vi "Save Data Single Station.vi"(5 "index":i32, 7 "Appliance Details":T1[](array[typedef]) {"Dryer"."Dryer Initial IMC Data"."Maximum Weight (lbf)" format="%03_6g"; "Dryer"."Dryer Initial IMC Data"."Average Weight (lbf)" format="%03_6g"; "Dryer"."Dryer Initial IMC Data"."Minimum Weight (lbf)" format="%03_6g"; "Dryer"."Dryer Initial IMC Data"."CEF (lbf/kWh)" format="%03_6g"; "Dryer"."Dryer Initial IMC Data"."Actual Final RMC (%)" format="%03_6g"; "Dryer"."Dryer Initial IMC Data"."Tolerance(%)" format="%0#_6g"; "Dryer"."Dryer Initial IMC Data"."Bone Dry Wt(lbs)" format="%03_6g"; "Dryer"."Dryer Initial IMC Data"."RMC (Desired %)" format="%0#_6g"; "Dryer"."Dryer Initial IMC Data"."Actual Initial RMC (%)" format="%03_6g"; "Dryer"."Dryer Initial IMC Data"."Measured IMC (lbs)" format="%0#_6g"}, 8 "Error In":errorcluster, 9 "File Locations in":T7, 10 "Data Array":string[][](array[string]), 11 "Log Data?":bool) -> (0 "Error Out":errorcluster, 2 "Saving":bool, 3 "File Locations out":T7)   [LabVIEW 2016]
uses:
  File Setup (Public)/Type Definition/Save File DOE File Path Control.ctl
  File Setup (Public)/Type Definition/Save File DOE Data Save Filepaths.ctl
  File Setup (Public)/Type Definition/Save File DISH Dishwasher Details.ctl
  <vilib>/Platform/fileVersionInfo.llb/FileVersionInformation.ctl
  Washer DOE/Type Definitions/DOE Appliance Common.ctl
  Custom Pallet Controls/Custom Pallet String.ctl
  File Setup (Public)/Type Definition/DPT IMC Data.ctl
  Washer DOE/Type Definitions/DOE Dryer Standard.ctl
  File Setup.lvlib
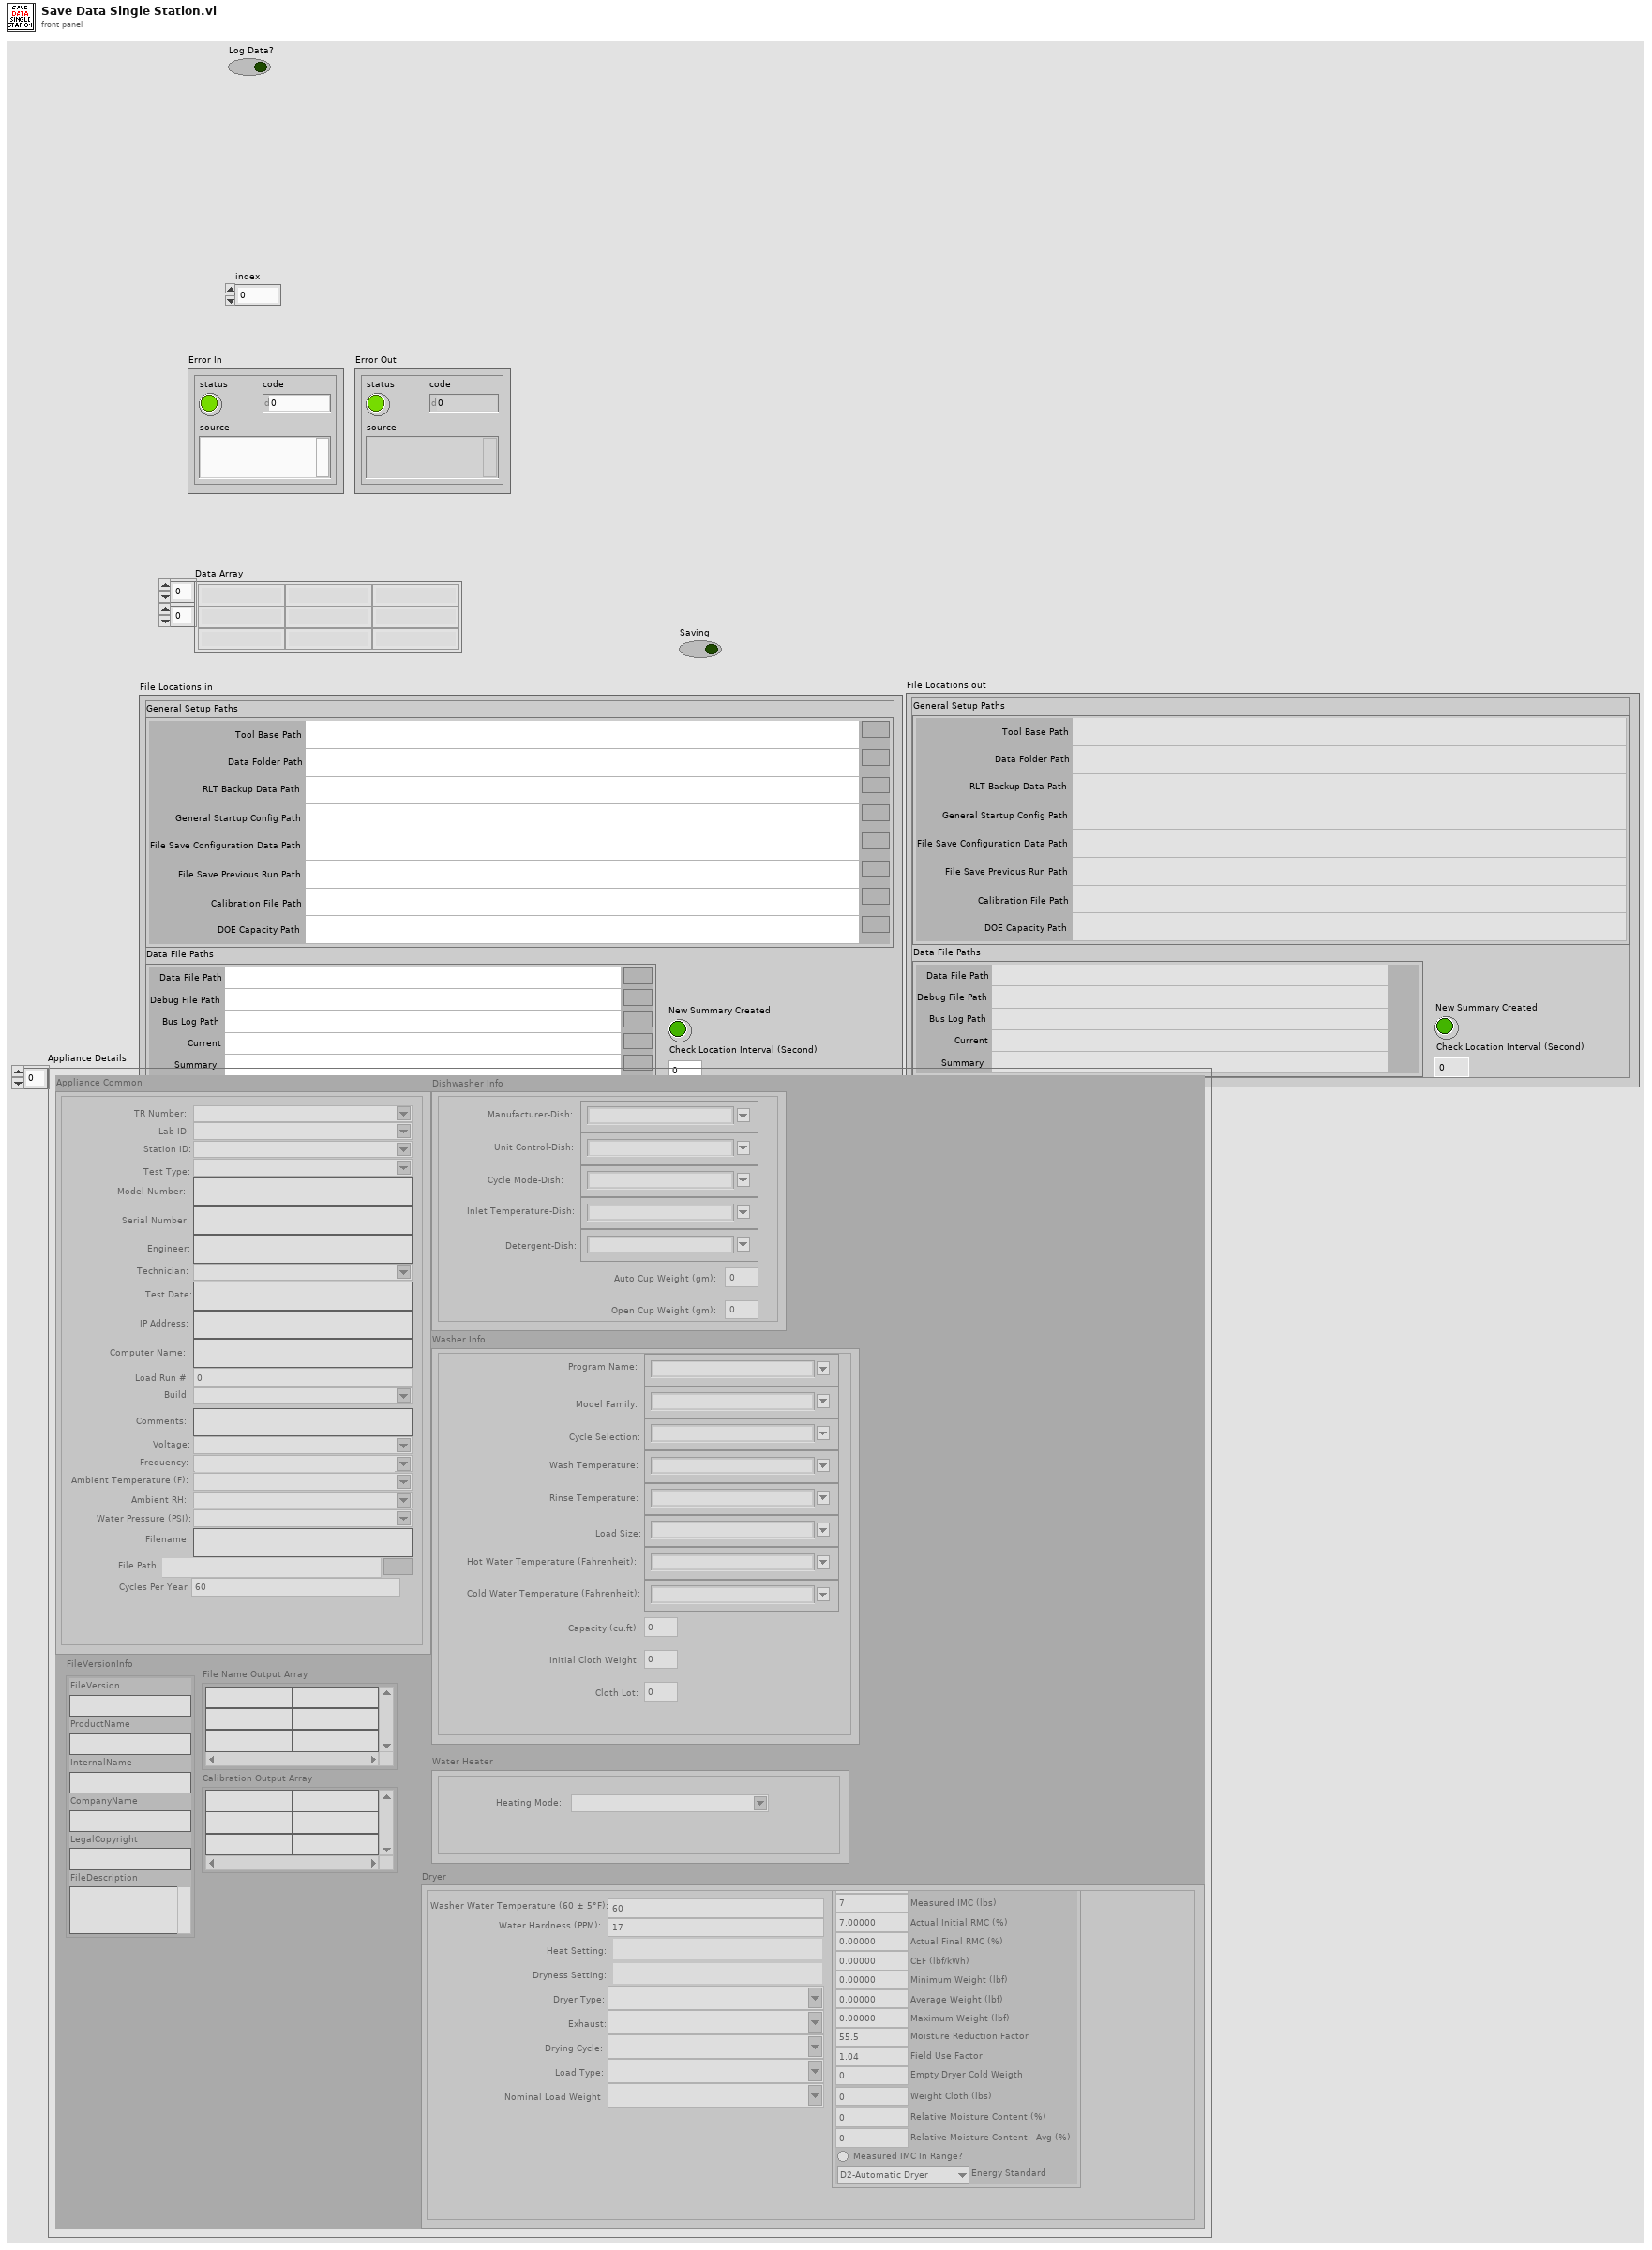
[diagram p1: front panel]
types:
  T1 = typedef "File Setup.lvlib/Save File DISH Dishwasher Details.ctl" = cluster{"FileVersionInfo":T2, "Dishwasher Info":cluster{"Open Cup Weight (gm):":dbl, "Auto Cup Weight (gm):":dbl, "Detergent-Dish:":string, "Inlet Temperature-Dish:":string, "Cycle Mode-Dish:":string, "Unit Control-Dish:":string, "Manufacturer-Dish:":string}, "Washer Info":cluster{"Hot Water Temperature (Fahrenheit):":string, "Cold Water Temperature (Fahrenheit):":string, "Capacity (cu.ft):":dbl, "Initial Cloth Weight:":dbl, "Cloth Lot:":i32, "Model Family:":string, "Program Name:":string, "Cycle Selection:":string, "Wash Temperature:":string, "Rinse Temperature:":string, "Load Size:":string}, "File Name Output Array":string[][], "Calibration Output Array":string[][], "Appliance Common":T3, "Water Heater":cluster{"Heating Mode:":string}, "Dryer":cluster{"Heat Setting:":T4, "Washer Water Temperature (60 ± 5°F):":u16, "Water Hardness (PPM):":u16, "Dryness Setting:":T4, "Dryer Type:":string, "Exhaust:":string, "Drying Cycle:":string, "Load Type:":string, "Nominal Load Weight":string, "Dryer Initial IMC Data":T5}}
  T2 = typedef "FileVersionInformation.ctl" = cluster{"FileVersion":string, "ProductName":string, "InternalName":string, "CompanyName":string, "LegalCopyright":string, "FileDescription":string}
  T3 = typedef "DOE Appliance Common.ctl" = cluster{"Engineer:":string, "Model Number:":string, "Serial Number:":string, "Comments:":string, "Station ID:":string, "Technician:":string, "TR Number:":string, "Lab ID:":string, "Voltage:":string, "Water Pressure (PSI):":string, "Test Date:":string, "Computer Name:":string, "IP Address:":string, "Ambient RH:":string, "Frequency:":string, "Build:":string, "Filename:":string, "Test Type:":string, "Load Run #:":i32, "Ambient Temperature (F):":string, "File Path:":path, "Cycles Per Year":u32}
  T4 = typedef "Custom Pallet String.ctl" = string
  T5 = typedef "DPT IMC Data.ctl" = cluster{"Measured IMC (lbs)":dbl, "Actual Initial RMC (%)":dbl, "RMC (Desired %)":dbl, "Bone Dry Wt(lbs)":dbl, "Tolerance(%)":dbl, "Actual Final RMC (%)":dbl, "CEF (lbf/kWh)":dbl, "Minimum Weight (lbf)":dbl, "Average Weight (lbf)":dbl, "Maximum Weight (lbf)":dbl, "Measured IMC In Range?":bool, "Moisture Reduction Factor":dbl, "Field Use Factor":dbl, "Empty Dryer Cold Weigth":dbl, "Energy Standard":T6, "Weight Cloth (lbs)":dbl, "Relative Moisture Content (%)":dbl, "Relative Moisture Content - Avg (%)":dbl}
  T6 = typedef "DOE Dryer Standard.ctl" = enum16{"D2-Automatic Dryer", "D2-Timer Dryer", "D1-Automatic Dryer", "D1-Timer Dryer", "Other"}
  T7 = typedef "File Setup.lvlib/Save File DOE File Path Control.ctl" = cluster{"General Setup Paths":cluster{"Calibration File Path":path, "DOE Capacity Path":path, "Data Folder Path":path, "RLT Backup Data Path":path, "Tool Base Path":path, "General Startup Config Path":path, "File Save Previous Run Path":path, "File Save Configuration Data Path":path}, "Data File Paths":T8, "New Summary Created":bool, "Check Location Interval (Second)":i32}
  T8 = typedef "File Setup.lvlib/Save File DOE Data Save Filepaths.ctl" = cluster{"Data File Path":path, "Debug File Path":path, "Bus Log Path":path, "Current":path, "Summary":path}
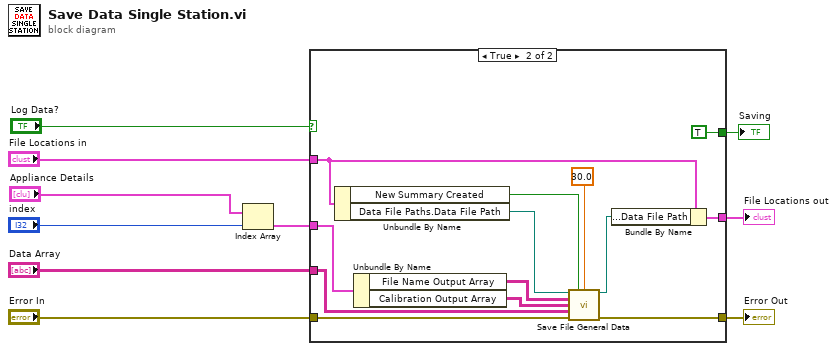
[diagram p0: block diagram]
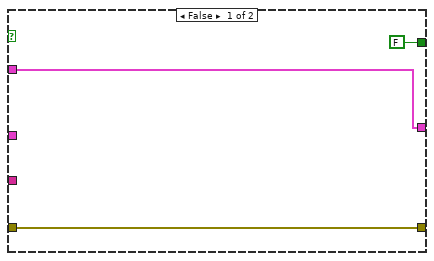
[diagram p2: hidden frame]
diagram:
  n1 = Index Array(array="Appliance Details", index="index") -> (element=w3:T1)
  n2 = case shown="True" "Log Data?" {
    tunnel: "Data Array" -> [_ w26]
    tunnel: [FALSE TRUE] -> w7
    tunnel: w3 -> [_ w23]
    tunnel: "File Locations in" -> [w12 w18]
    tunnel: [w12 w17] -> w10
    tunnel: "Error In" -> [w11 w16]
    tunnel: [w11 w15] -> w5
    frame False {
    }
    frame True {
      n3 = Unbundle By Name(w18) -> ("New Summary Created"=w19:bool, "Data File Paths.Data File Path"=w14:path)
      n4 = Unbundle By Name(w23) -> ("File Name Output Array"=w22:string[][], "Calibration Output Array"=w21:string[][])
      n5 = call "Save File General Data.vi"("Data File Path In"=w14, "New File (Path Change)"=w19, "File Size"=30.0, "File Name Output Array"=w22, "Calibration Output Array"=w21, "Save Data"=w26, "Error In"=w16) -> ("Data File Path Out"=w20:path, "Error Out"=w15:errorcluster)  [unwired: 6 in, 1 out]
      n6 = Bundle By Name(cluster=w18, "Data File Paths.Data File Path"=w20) -> (w17:T7)
    }
  }
  "File Locations out" <- w10
  "Saving" <- w7
  "Error Out" <- w5
